vi "Keyboard & Graphs.vi"() -> ()   [LabVIEW 2014]
doc: "Very simple example showing how to use the base VIs to control the AR Drone and receive and display navigation data."
uses:
  <vilib>/LVH/AR Drone Toolkit/Decode NavData/Typedefs/NavData Demo.ctl
  <vilib>/LVH/AR Drone Toolkit/AR Drone.lvlib
panel:
  out "error out 2":errorcluster
  out "error out":errorcluster
  out "NavData Out":T1={"control state"=enum."TRANS_LANDING", "battery percentage"=33, "pitch (deg)"=0.507, "roll (deg)"=-0.212, "yaw (deg)"=116.625, "altitude (cm)"=0, "vx (cm/s)?"=0.0, "vy (cm/s)?"=0.0, "vz (cm/s)?"=0.0, "detection cam type"=3}
  out "Battery Remaining":dbl(slide)=33.0 scale=0.0..100.0
  out "Tilt":T2(graph)={"pitch (deg)"=0.507, "roll (deg)"=-0.212, "yaw (deg)"=116.625}
  out "Altitude":u32(graph)
  out "vy":sgl(graph)
  out "vx":sgl(graph)
  in  "Speed value":dbl=0.01
  out "Control cluster":T3 {"Roll" scale=-1.0..1.0; "Pitch" scale=-1.0..1.0; "Vertical Speed" scale=-1.0..1.0; "Yaw Speed" scale=-1.0..1.0}
  in  "stop":bool
  in  "Emergency Landing":bool
  in  "Take Off/Land":bool
  in  "Hover":bool
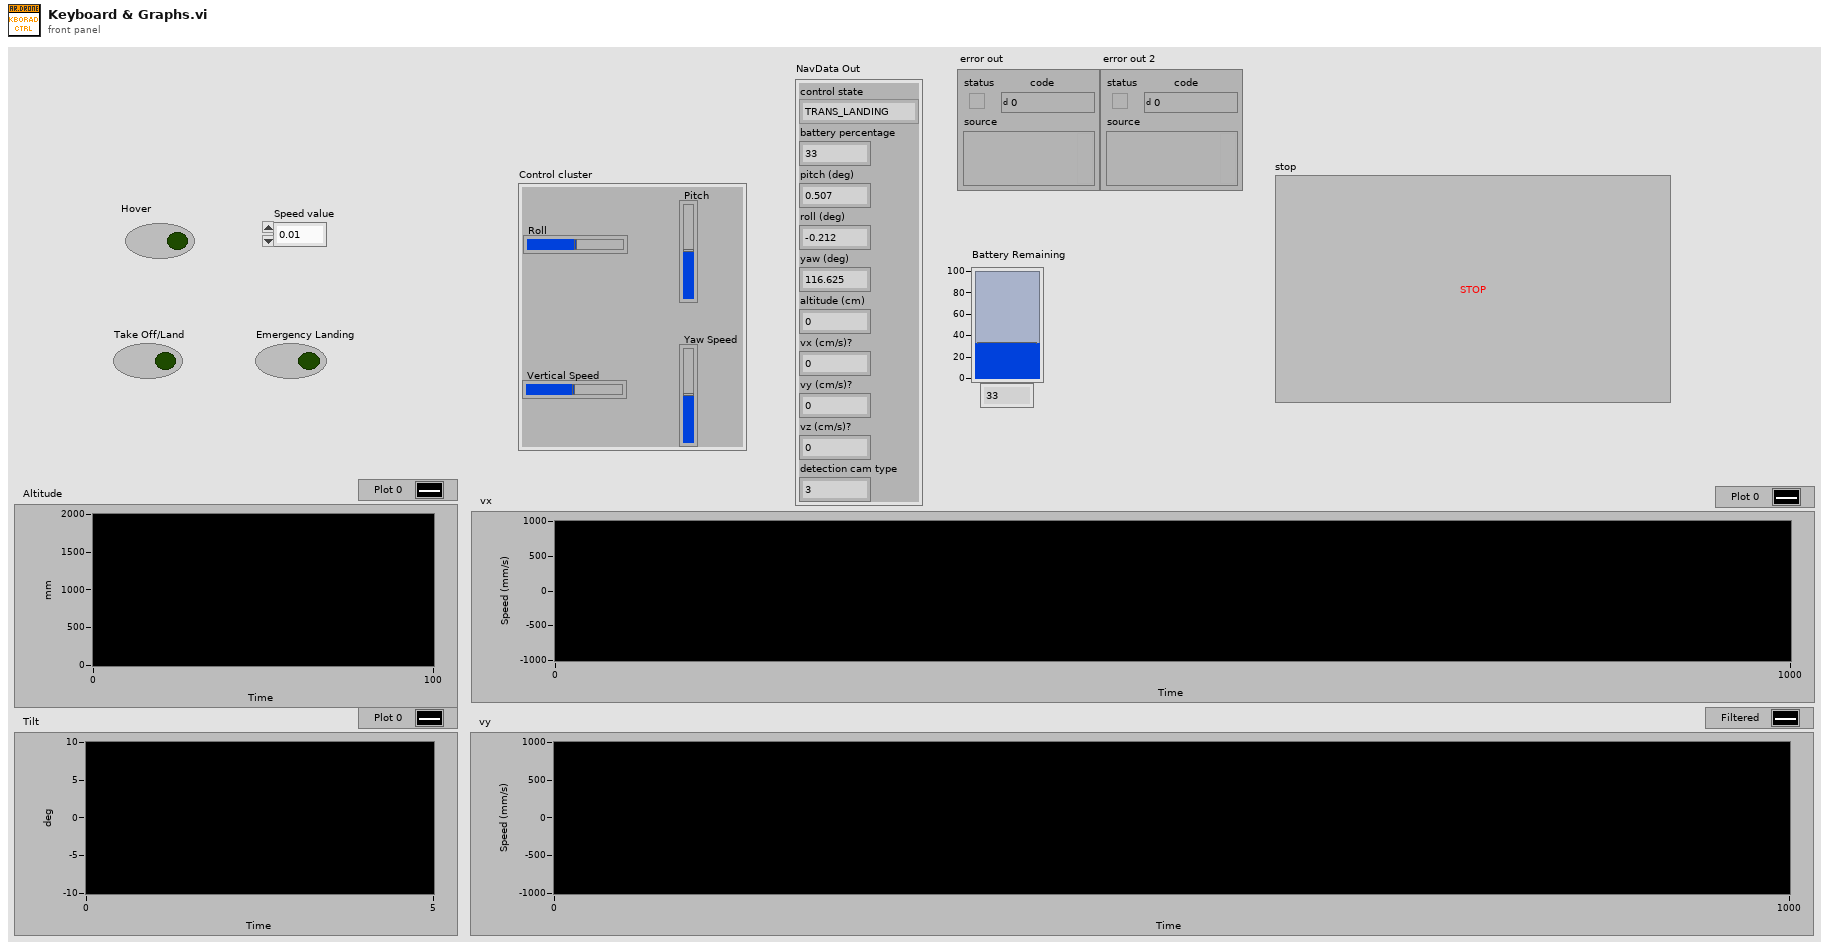
[diagram p1: front panel]
types:
  T1 = typedef "AR Drone.lvlib/NavData Demo.ctl" = cluster{"control state":enum32{"DEFAULT", "INIT", "LANDING", "FLYING", "HOVERING", "TEST", "TRANS_TAKEOFF", "TRANS_GOTOFIX", "TRANS_LANDING"}, "battery percentage":u32, "pitch (deg)":sgl, "roll (deg)":sgl, "yaw (deg)":sgl, "altitude (cm)":u32, "vx (cm/s)?":sgl, "vy (cm/s)?":sgl, "vz (cm/s)?":sgl, "detection cam type":u32}
  T2 = cluster{"pitch (deg)":sgl, "roll (deg)":sgl, "yaw (deg)":sgl}
  T3 = cluster{"Roll":dbl, "Pitch":dbl, "Vertical Speed":dbl, "Yaw Speed":dbl}
  T4 = typedef "AR Drone.lvlib/AR Drone Resource.ctl" = cluster{"UDP Control Connection":refnum<k16>, "UDP NavData Connection":refnum<k16>, "UDP Video Connection (Drone 1.0)":refnum<k16>, "TCP Video Connection (Drone 2.0)":refnum<k5>, "TCP Control Port Connection":refnum<k5>, "Drone IP address":string, "Drone Command Port":u16, "Drone NavData Port":u16, "Drone Vid Stream Port":u16, "Drone TCP Control Port":u16, "Home IP address":string, "Home Command Port":u16, "Home NavData Port":u16, "Home Vid Stream Port":u16, "Drone Version":i32, "Drone Index":i32, "Command Sequence":i32}
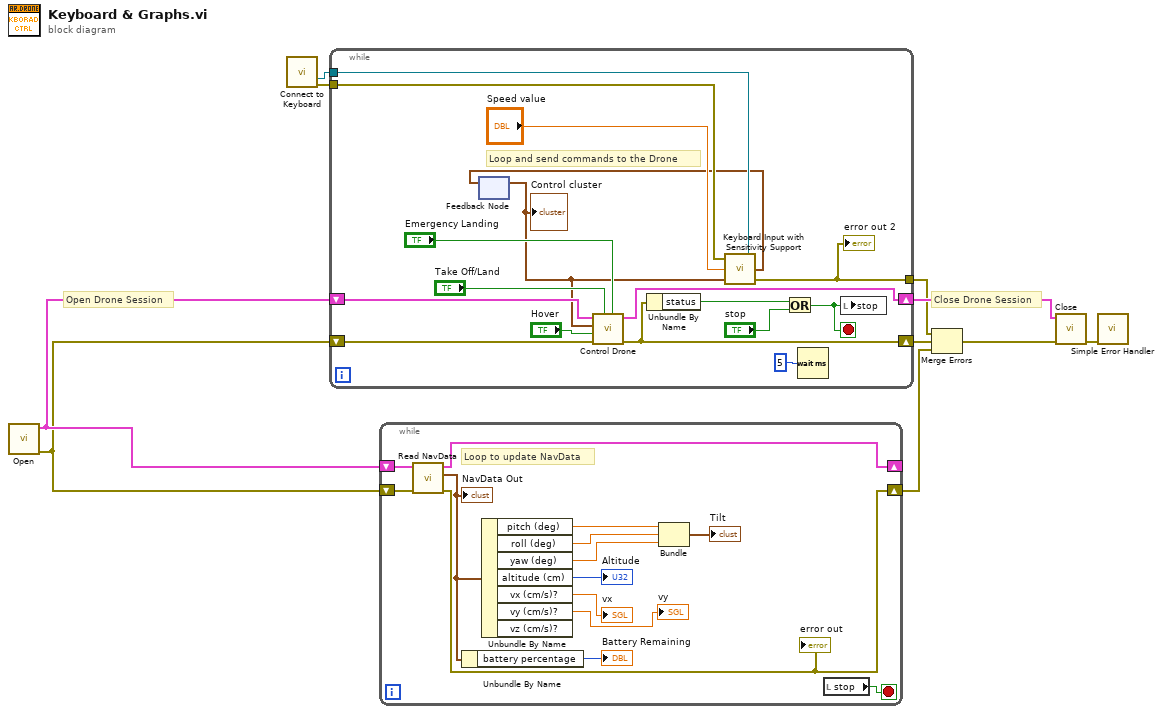
[diagram p0: block diagram]
diagram:
  # "Close Drone Session"
  # "Open Drone Session"
  n1 = call <vilib>:"Open.vi"() -> ("error out"=w2:errorcluster, "AR Drone Resource"=w3:T4)  [unwired: 10 in]
  n2 = call "Connect to Keyboard.vi"() -> ("device ID"=w5:refnum<k1>, "error out"=w6:errorcluster)  [unwired: 13 in, 1 out]
  n3 = while {
    shift-right: [w22] -> w10
    shift-left: w3 -> [w26]
    shift-right: [w18] -> w7
    shift-left: w2 -> [w27]
    tunnel: w6 -> [w15]
    tunnel: [w11] -> w4
    tunnel: w5 -> [w16]
    stop <- w17 stop-if-true
    # "Loop and send commands to the Drone"
    n4 = feedback #1() -> (w12:T3)  [unwired: 1 in]
    "Control cluster" <- w12
    n5 = call <vilib>:"Control Drone.vi"("Emergency Landing"="Emergency Landing", "Takeoff/Land"="Take Off/Land", "error in (no error)"=w27, "Hover"="Hover", "Control Cluster"=w12, "AR Drone Resource"=w26) -> ("error out"=w18:errorcluster, "AR Drone Resource Out"=w22:T4)  [unwired: 4 in]
    n6 = Unbundle By Name(w18) -> ("status"=w20:bool)
    n7 = call "Keyboard Input with Sensitivity Support.vi"("device ID"=w16, "Previous Control Cluster"=w12, "Speed step"="Speed value", "error in (no error)"=w15) -> ("error out"=w11:errorcluster, "Control Cluster"=w13:T3)
    "error out 2" <- w11
    n8 = feedback-in #1(w13) -> ()
    n9 = Or(x=w20, y="stop") -> (x .or. y?=w17:bool)
    n10 = Wait (ms)(milliseconds to wait=u32 5) -> ()  [unwired: 1 out]
    n11 = local write "stop"(w17) -> ()
  }
  n12 = while {
    shift-right: [w39] -> _
    shift-left: w3 -> [w40]
    shift-right: [w37] -> w1
    shift-left: w2 -> [w38]
    stop <- w41 stop-if-true
    # "Loop to update NavData"
    n13 = call <vilib>:"Read NavData.vi"("error in (no error)"=w38, "AR Drone Resource"=w40) -> ("error out"=w37:errorcluster, "NavData Out"=w35:T1, "AR Drone Resource Out"=w39:T4)  [unwired: 7 in]
    "NavData Out" <- w35
    "error out" <- w37
    n14 = Unbundle By Name(w35) -> ("battery percentage"=→"Battery Remaining":u32)
    n15 = Unbundle By Name(w35) -> ("pitch (deg)"=w31:sgl, "roll (deg)"=w34:sgl, "yaw (deg)"=w33:sgl, "altitude (cm)"=→"Altitude":u32, "vx (cm/s)?"=→"vx":sgl, "vy (cm/s)?"=→"vy":sgl)  [unwired: 1 out]
    n16 = Bundle("pitch (deg)"=w31, "roll (deg)"=w34, "yaw (deg)"=w33) -> (→"Tilt":T2)  [unwired: 1 in]
    n17 = local read "stop"() -> (w41:bool)
  }
  n18 = Merge Errors(w4, w7, w1) -> (w8:errorcluster)
  n19 = call <vilib>:"Close.vi"("error in (no error)"=w8, "AR Drone Resource"=w10) -> ("error out"=w9:errorcluster)  [unwired: 9 in]
  n20 = call <vilib>:"Simple Error Handler.vi"("error in (no error)"=w9) -> ()  [unwired: 4 in, 5 out]
